vi "Send Message To Execution Engine.vi"(0 "Message":string, 5 "Message Type":i32(ring) items=["Info", "Warning", "Error", "Action"], 11 "error in":errorcluster) -> (15 "error out":errorcluster)   [LabVIEW 2023, in "RFFixtureCharact.Public.lvlib"]
uses:
  RFFixtureCharact.Public.lvlib
  Common/RFCalAndFixtureCharact.Common.lvlib
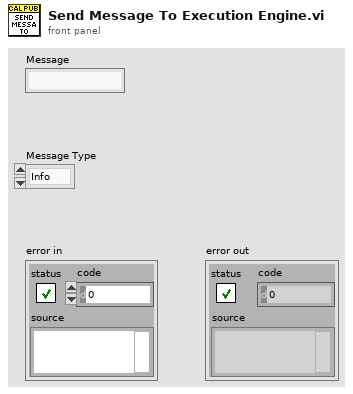
[diagram p1: front panel]
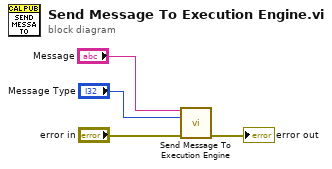
[diagram p0: block diagram]
diagram:
  n1 = call "Send Message To Execution Engine.vi"("Message"="Message", "Message Type"="Message Type", "error in (no error)"="error in") -> ("error out"=→"error out":errorcluster)  [unwired: 12 in]
